vi "Release.vi"() -> ()   [LabVIEW 2024]
uses:
  C:/Users/Andrey/Desktop/wpf_in_trouble/LVtest/WindowsFormsControlLibrary.dll
  WindowsFormsControlLibrary.dll
panel:
  in  "UserControl1":refnum<k24>(container)
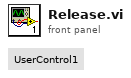
[diagram p1: front panel]
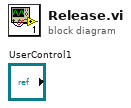
[diagram p0: block diagram]
diagram:
